vi "Field to Pixel.vi"(8 "Field Coordinate Y":dbl, 10 "Field Coordinate X":dbl) -> (0 "Pixel Y":dbl, 2 "Pixel X":dbl)   [LabVIEW 2013]
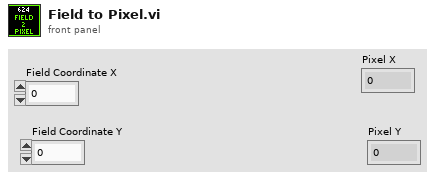
[diagram p1: front panel]
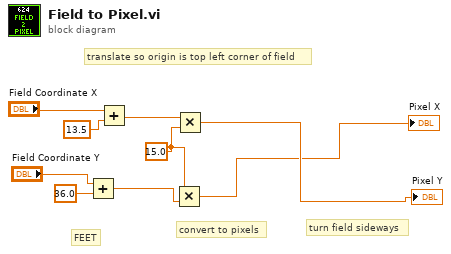
[diagram p0: block diagram]
diagram:
  w3 = 15.0 ("y")
  # "turn field sideways"
  # "convert to pixels"
  # "FEET"
  # "translate so origin is top left corner of field"
  n1 = Add(x="Field Coordinate Y", y=36.0) -> (x+y=w4:dbl)
  n2 = Add(x="Field Coordinate X", y=13.5) -> (x+y=w5:dbl)
  n3 = Multiply(x=w3, y=w4) -> (x*y=→"Pixel X":dbl)
  n4 = Multiply(x=w5, y=w3) -> (x*y=→"Pixel Y":dbl)
